vi "Fault_Table_Read.vi"(7 "ERD Data Out":T3[](array[typedef]) {"ERD Number" format="%.0x"}) -> (1 "Fault Set?":bool, 2 "Table Buffer Status":T4, 3 "Fault Table String Out":string[][](array[string]), 4 "Fault Table Array Out":T1)   [LabVIEW 2016]
uses:
  type defs/Fault_Buffer_Status.ctl
  Common/LabVIEW GEA2 Toolkit/LabVIEW_GEA2_Toolkit.lvlibp/type defs/ERD Read Data Out.ctl
  Laundry Tool 2.0 Support/type defs2/Fault Table Array.ctl
  type defs/Fault_Table_Info.ctl
  Common/LabVIEW GEA2 Toolkit/LabVIEW_GEA2_Toolkit.lvlibp
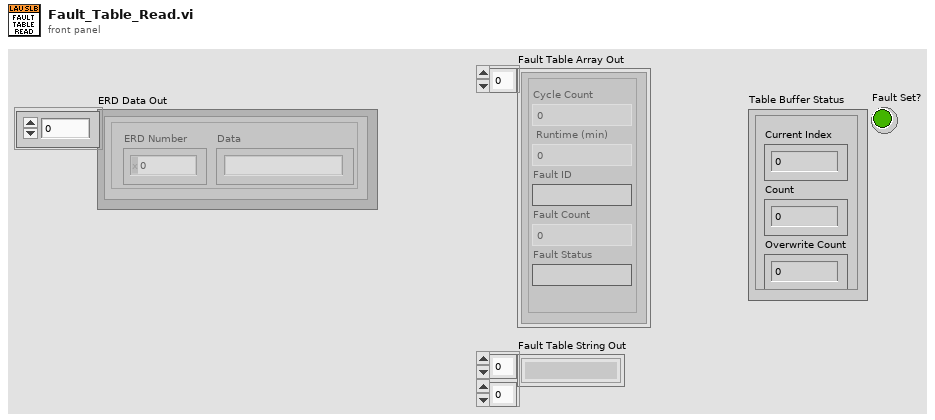
[diagram p1: front panel]
types:
  T1 = typedef "Fault Table Array.ctl" = T2[]
  T2 = typedef "Fault_Table_Info.ctl" = cluster{"Cycle Count":u32, " Runtime (min) ":u32, "Fault Status":string, "Fault ID":string, "Fault Count":u16}
  T3 = typedef "LabVIEW_GEA2_Toolkit.lvlibp/ERD Read Data Out.ctl" = cluster{"ERD Number":u16, "Data":string}
  T4 = typedef "Fault_Buffer_Status.ctl" = cluster{"Current Index":u16, "Count":u16, "Overwrite Count":u16}
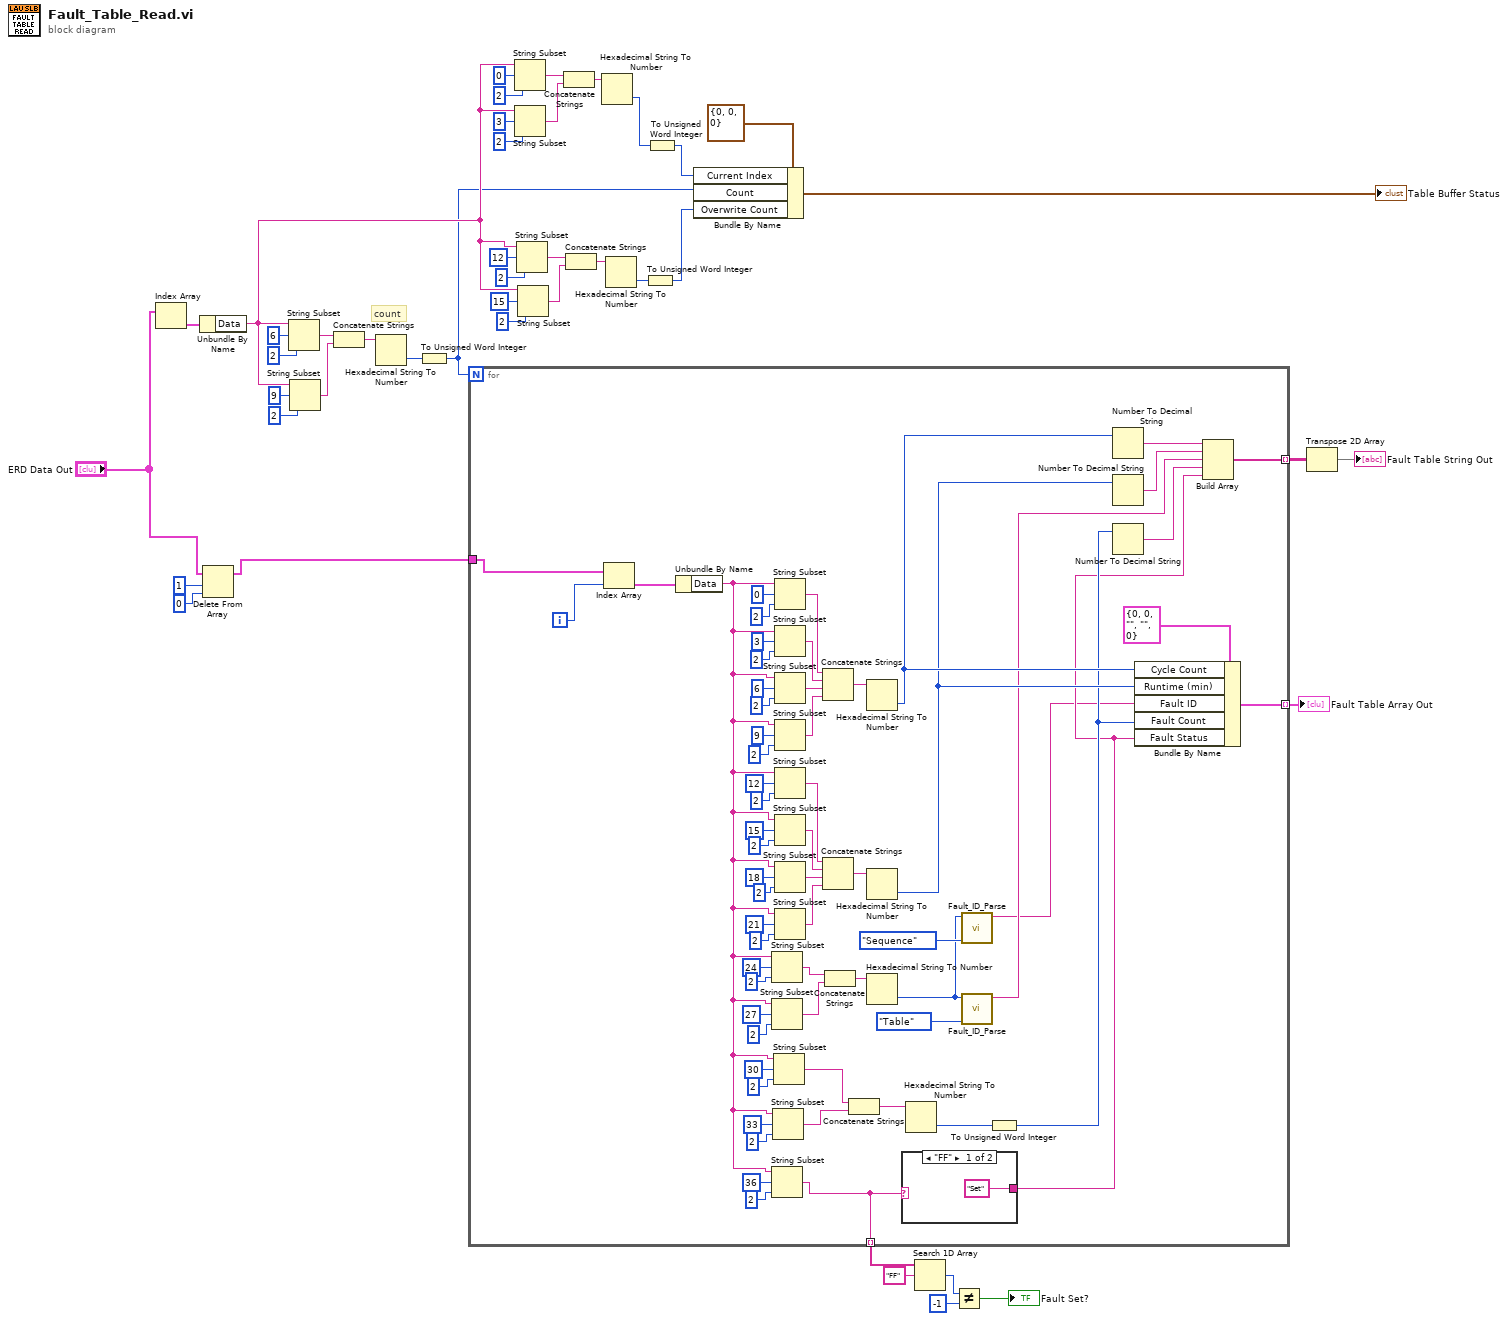
[diagram p0: block diagram]
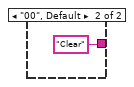
[diagram p2: hidden frame]
diagram:
  # "count"
  n1 = Index Array(array="ERD Data Out") -> (element=w36:T3)  [unwired: 1 in]
  n2 = Unbundle By Name(w36) -> ("Data"=w15:string)
  n3 = Delete From Array(array="ERD Data Out", length=1, index=0) -> (array with subset deleted=w5:T3[])  [unwired: 1 out]
  n4 = String Subset(string=w15, offset (0)=6, length (rest)=2 ("length (rest)")) -> (substring=w40:string)
  n5 = String Subset(string=w15, offset (0)=9, length (rest)=2 ("length (rest)")) -> (substring=w39:string)
  n6 = Concatenate Strings(w40, w39) -> (w38:string)
  n7 = Hexadecimal String To Number(string=w38) -> (number=w37:u32)  [unwired: 2 in, 1 out]
  n8 = To Unsigned Word Integer(number=w37) -> (unsigned 16bit integer=w8:u16)
  n9 = for {
    N: w8 -> [_]
    tunnel: [w61] -> w1 mode=indexing
    tunnel: [w59] -> w13 mode=indexing
    tunnel: w5 -> [w57]
    tunnel: [w48] -> w3 mode=indexing
    i -> [w58]
    n10 = Index Array(array=w57, index=w58) -> (element=w60:T3)
    n11 = Unbundle By Name(w60) -> ("Data"=w66:string)
    n12 = String Subset(string=w66, offset (0)=24, length (rest)=2 ("length (rest)")) -> (substring=w85:string)
    n13 = String Subset(string=w66, offset (0)=27, length (rest)=2 ("length (rest)")) -> (substring=w84:string)
    n14 = String Subset(string=w66, offset (0)=36, length (rest)=2 ("length (rest)")) -> (substring=w59:string)
    n15 = String Subset(string=w66, offset (0)=33, length (rest)=2 ("length (rest)")) -> (substring=w63:string)
    n16 = String Subset(string=w66, offset (0)=30, length (rest)=2 ("length (rest)")) -> (substring=w64:string)
    n17 = String Subset(string=w66, offset (0)=0, length (rest)=2 ("length (rest)")) -> (substring=w101:string)
    n18 = String Subset(string=w66, offset (0)=3, length (rest)=2 ("length (rest)")) -> (substring=w100:string)
    n19 = String Subset(string=w66, offset (0)=6, length (rest)=2 ("length (rest)")) -> (substring=w99:string)
    n20 = String Subset(string=w66, offset (0)=9, length (rest)=2 ("length (rest)")) -> (substring=w98:string)
    n21 = String Subset(string=w66, offset (0)=12, length (rest)=2 ("length (rest)")) -> (substring=w92:string)
    n22 = String Subset(string=w66, offset (0)=15, length (rest)=2 ("length (rest)")) -> (substring=w93:string)
    n23 = String Subset(string=w66, offset (0)=18, length (rest)=2 ("length (rest)")) -> (substring=w94:string)
    n24 = String Subset(string=w66, offset (0)=21, length (rest)=2 ("length (rest)")) -> (substring=w95:string)
    n25 = Concatenate Strings(w101, w100, w99, w98) -> (w97:string)
    n26 = Concatenate Strings(w92, w93, w94, w95) -> (w96:string)
    n27 = Concatenate Strings(w85, w84) -> (w83:string)
    n28 = Concatenate Strings(w64, w63) -> (w65:string)
    n29 = Hexadecimal String To Number(string=w97) -> (number=w56:u32)  [unwired: 2 in, 1 out]
    n30 = Hexadecimal String To Number(string=w96) -> (number=w55:u32)  [unwired: 2 in, 1 out]
    n31 = Hexadecimal String To Number(string=w83) -> (number=w45:u32)  [unwired: 2 in, 1 out]
    n32 = case shown="\"FF\"" w59 {
      tunnel: ["Set" "Clear"] -> w49
      frame "FF" {
      }
      frame "00", Default {
      }
    }
    n33 = Hexadecimal String To Number(string=w65) -> (number=w62:u32)  [unwired: 2 in, 1 out]
    n34 = call "Fault_ID_Parse.vi"("Enum"=enum16{"Sequence", "Table"}."Sequence", "Numeric"=w45) -> ("String"=w44:string)  [unwired: 9 in]
    n35 = call "Fault_ID_Parse.vi"("Enum"=enum16{"Sequence", "Table"}."Table", "Numeric"=w45) -> ("String"=w51:string)  [unwired: 9 in]
    n36 = To Unsigned Word Integer(number=w62) -> (unsigned 16bit integer=w54:u16)
    n37 = Number To Decimal String(number=w56) -> (decimal integer string=w53:string)  [unwired: 1 in]
    n38 = Number To Decimal String(number=w55) -> (decimal integer string=w52:string)  [unwired: 1 in]
    n39 = Number To Decimal String(number=w54) -> (decimal integer string=w50:string)  [unwired: 1 in]
    n40 = Bundle By Name(cluster=T2 {"Cycle Count"=0, " Runtime (min) "=0, "Fault Status"="", "Fault ID"="", "Fault Count"=0} ("Fault Table 0"), "Cycle Count"=w56, "Runtime (min)"=w55, "Fault ID"=w44, "Fault Count"=w54, "Fault Status"=w49) -> (w61:T2)
    n41 = Build Array(w53, w52, w51, w50, w49) -> (w48:string[])
  }
  "Fault Table Array Out" <- w1
  n42 = String Subset(string=w15, offset (0)=0, length (rest)=2 ("length (rest)")) -> (substring=w24:string)
  n43 = String Subset(string=w15, offset (0)=3, length (rest)=2 ("length (rest)")) -> (substring=w25:string)
  n44 = String Subset(string=w15, offset (0)=12, length (rest)=2 ("length (rest)")) -> (substring=w26:string)
  n45 = String Subset(string=w15, offset (0)=15, length (rest)=2 ("length (rest)")) -> (substring=w27:string)
  n46 = Concatenate Strings(w24, w25) -> (w28:string)
  n47 = Concatenate Strings(w26, w27) -> (w29:string)
  n48 = Hexadecimal String To Number(string=w28) -> (number=w31:u32)  [unwired: 2 in, 1 out]
  n49 = Hexadecimal String To Number(string=w29) -> (number=w32:u32)  [unwired: 2 in, 1 out]
  n50 = To Unsigned Word Integer(number=w32) -> (unsigned 16bit integer=w34:u16)
  n51 = To Unsigned Word Integer(number=w31) -> (unsigned 16bit integer=w33:u16)
  n52 = Bundle By Name(cluster=T4 {"Current Index"=0, "Count"=0, "Overwrite Count"=0} ("Buffer Status"), "Current Index"=w33, "Count"=w8, "Overwrite Count"=w34) -> (→"Table Buffer Status":T4)
  n53 = Search 1D Array(1D array=w13, element="FF") -> (index of element=w11:i32)  [unwired: 1 in]
  n54 = Not Equal?(x=w11, y=-1) -> (x != y?=→"Fault Set?":bool)
  n55 = Transpose 2D Array(2D array=w3) -> (transposed array=→"Fault Table String Out":string[][])
